vi "Plot resize vertical.vi"(8 "error in (no error)":errorcluster, 11 "Refs":T1) -> (0 "error out":errorcluster, 2 "#rows hidden":u32, 3 "#rows visible":u32)   [LabVIEW 2021, in "RocketPlot.lvlib"]
uses:
  RocketPlot.lvlib
  TypeDefs/Plot UI references.ctl
  Classes/RocketPlotHandle/RocketPlotHandle.lvclass
  <userlib>/bjustice/TipStripOOPanel/Classes/TipPanelHandle/TipPanelHandle.lvclass
  TypeDefs/Plot top row.ctl
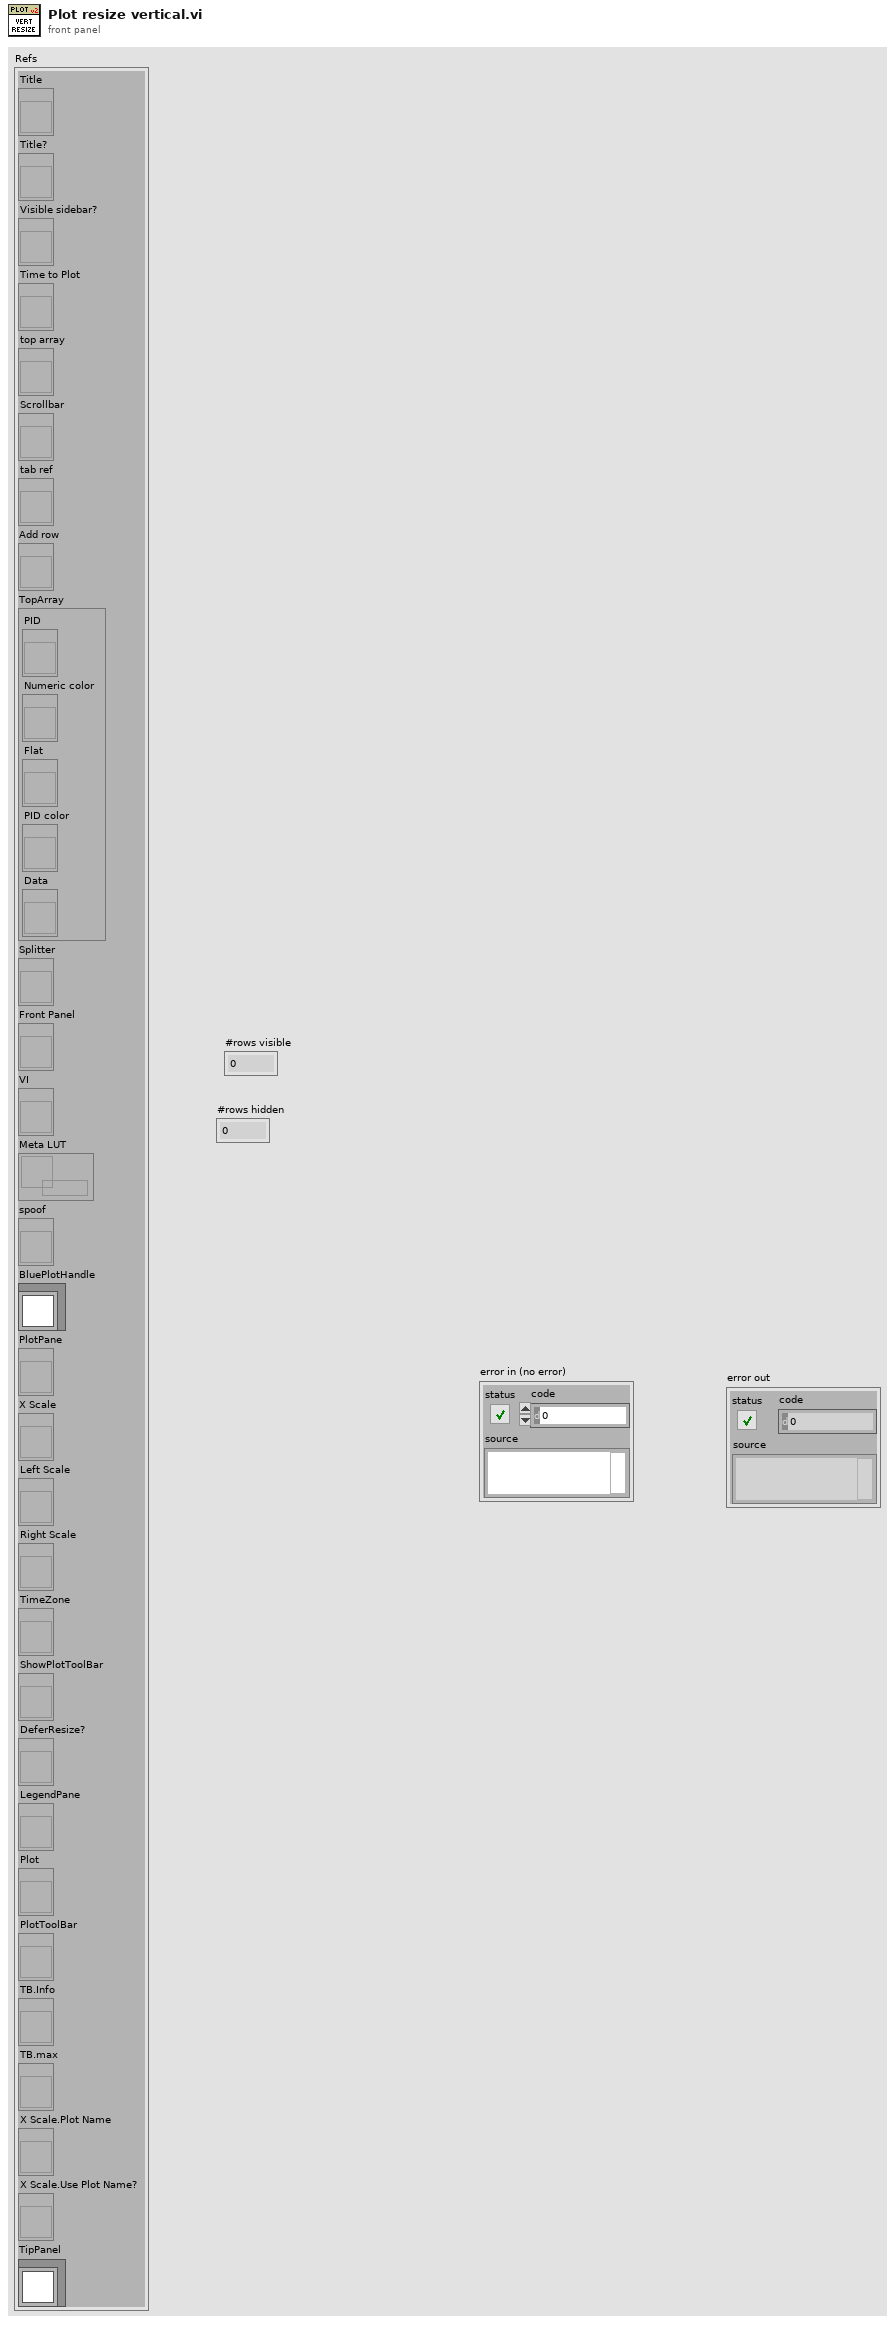
[diagram p1: front panel]
types:
  T1 = typedef "RocketPlot.lvlib/Plot UI references.ctl" = cluster{"Title":refnum<vi>, "Title?":refnum<vi>, "Visible sidebar?":refnum<vi>, "Time to Plot":refnum<vi>, "top array":refnum<vi>, "Scrollbar":refnum<vi>, "tab ref":refnum<vi>, "Add row":refnum<vi>, "TopArray":cluster{"PID":refnum<vi>, "Numeric color":refnum<vi>, "Flat":refnum<vi>, "PID color":refnum<vi>, "Data":refnum<vi>}, "Splitter":refnum<vi>, "Front Panel":refnum<vi>, "VI":refnum<vi>, "Meta LUT":refnum<data-value>, "spoof":refnum<vi>, "BluePlotHandle":refnum<class "RocketPlotHandle.lvclass">, "PlotPane":refnum<vi>, "X Scale":refnum<vi>, "Left Scale":refnum<vi>, "Right Scale":refnum<vi>, "TimeZone":refnum<vi>, "ShowPlotToolBar":refnum<vi>, "DeferResize?":refnum<vi>, "LegendPane":refnum<vi>, "Plot":refnum<vi>, "PlotToolBar":refnum<vi>, "TB.Info":refnum<vi>, "TB.max":refnum<vi>, "X Scale.Plot Name":refnum<vi>, "X Scale.Use Plot Name?":refnum<vi>, "TipPanel":refnum<class "TipPanelHandle.lvclass">}
  T2 = typedef "Plot top row.ctl" = cluster{"PID":string, "index":i32, "PID color":u32, "right axis?":bool, "Flatline?":bool, "Numeric color":u32, "Data":string, "Flat":string}
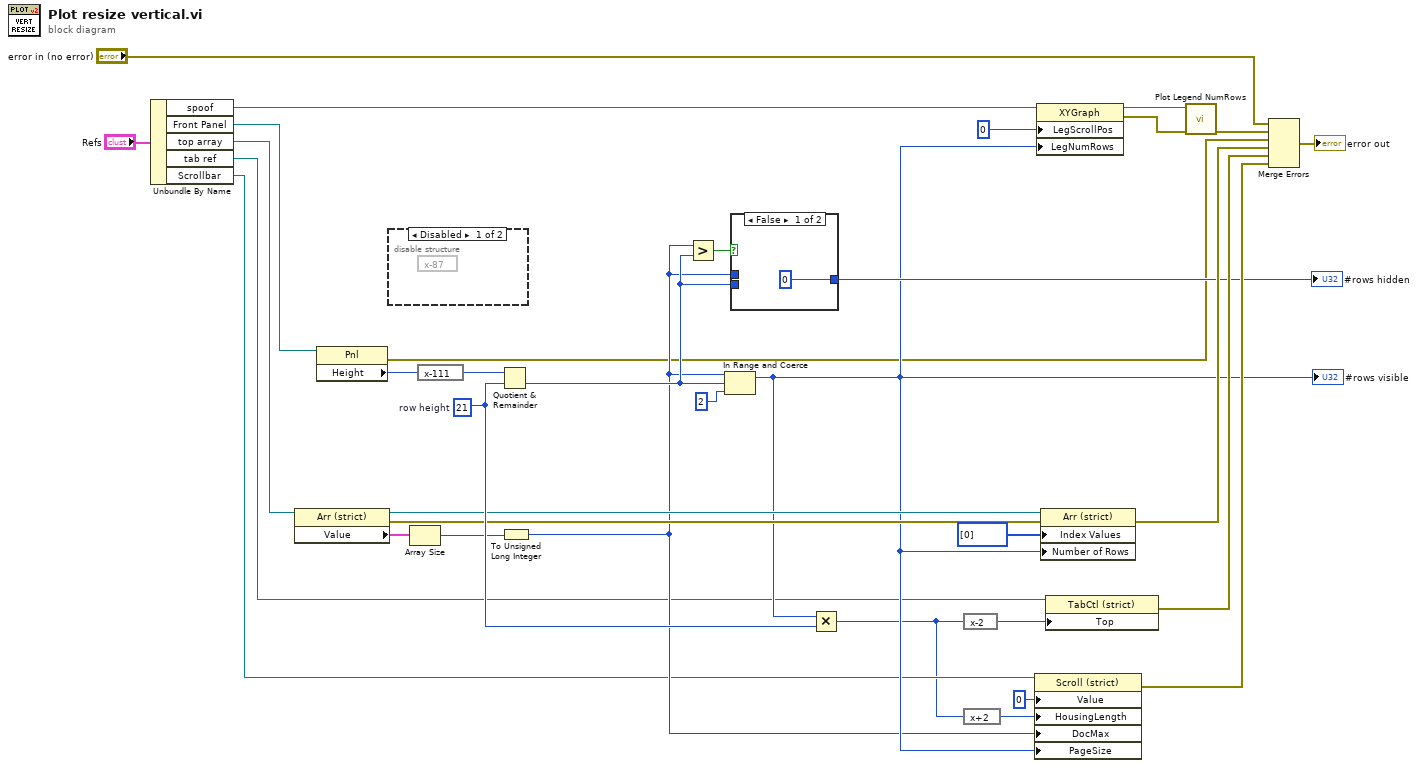
[diagram p0: block diagram]
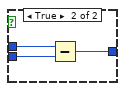
[diagram p3: hidden frame]
diagram:
  w29 = u32 21  # row height
  n1 = Unbundle By Name("Refs") -> ("spoof"=w9:refnum<vi>, "Front Panel"=w5:refnum<vi>, "top array"=w8:refnum<vi>, "tab ref"=w7:refnum<vi>, "Scrollbar"=w6:refnum<vi>)
  n2 = property on="Property Node" class="Arr (strict)"(reference=w8) -> (reference out=w19:refnum<vi>, error out=w18:errorcluster, "Value"=w20:T2[])  [unwired: 1 in]
  n3 = property class="Pnl"(reference=w5) -> (error out=w3:errorcluster, "Height"=w4:u32)  [unwired: 1 in, 1 out]
  n4 = disable-structure shown="Disabled" {
    frame Disabled {
      n5 = expression code="x-87"() -> ()  [unwired: 1 in, 1 out]
    }
    frame Enabled {
    }
  }
  n6 = Array Size(array=w20) -> (size(s)=w16:i32)
  n7 = expression code="x-111"(w4) -> (w34:u32)
  n8 = Quotient & Remainder(x=w34, y=w29) -> (floor(x/y)=w14:u32)  [unwired: 1 out]
  n9 = To Unsigned Long Integer(number=w16) -> (unsigned 32bit integer=w11:u32)
  n10 = Greater?(x=w11, y=w14) -> (0:w15:bool)
  n11 = In Range and Coerce(upper limit=w11, x=w14, lower limit=u32 2) -> (coerced(x)=w12:u32)  [unwired: 1 out]
  "#rows visible" <- w12
  n12 = case shown="False" w15 {
    tunnel: w11 -> [_ w38]
    tunnel: w14 -> [_ w37]
    tunnel: [u32 0 w36] -> w13
    frame False {
    }
    frame True {
      n13 = Subtract(x=w38, y=w37) -> (x-y=w36:u32)
    }
  }
  "#rows hidden" <- w13
  n14 = Multiply(x=w12, y=w29) -> (x*y=w2:u32)
  n15 = expression code="x-2"(w2) -> (w28:u32)
  n16 = expression code="x+2"(w2) -> (w1:u32)
  n17 = property on="Property Node" class="Scroll (strict)"(reference=w6, "Value"=0, "HousingLength"=w1, "DocMax"=w11, "PageSize"=w12) -> (error out=w22:errorcluster)  [unwired: 1 in, 1 out]
  n18 = property class="XYGraph"(reference=w9, "LegScrollPos"=u32 0 ("Legend:Scroll Position"), "LegNumRows"=w12) -> (reference out=w30:refnum<vi>, error out=w26:errorcluster)  [unwired: 1 in]
  n19 = property on="Property Node" class="Arr (strict)"(reference=w19, error in=w18, "Index Values"=u32[] [0], "Number of Rows"=w12) -> (error out=w24:errorcluster)  [unwired: 1 out]
  n20 = property on="Property Node" class="TabCtl (strict)"(reference=w7, "Top"=w28) -> (error out=w23:errorcluster)  [unwired: 1 in, 1 out]
  n21 = call "Plot Legend NumRows.vi"("error in (no error)"=w26, "XY graph ref"=w30) -> ("error out"=w25:errorcluster)  [unwired: 8 in, 1 out]
  n22 = Merge Errors("error in (no error)", w25, w3, w24, w23, w22) -> (→"error out":errorcluster)
